vi "Add User.vi"(8 "error in (no error)":errorcluster, 9 "Data":T1={"Password"="", "Access"=enum."Guest", "Array of Permissions"=[]}, 10 "Username":string, 11 "UserPwd DB in":refnum<class "UserPwd DB.lvclass">) -> (0 "error out":errorcluster, 3 "UserPwd DB out":refnum<class "UserPwd DB.lvclass">)   [LabVIEW 2016, in "UserPwd DB.lvlib" / "UserPwd DB.lvclass"]
uses:
  <userlib>/Common Components/UserPwd DB/UserPwd DB/UserPwd DB.lvclass
  <userlib>/Common Components/UserPwd DB/UserPwd DB/Data input.ctl
  <userlib>/Common Components/UserPwd DB/UserPwd DB/Access Level.ctl
  <userlib>/Common Components/UserPwd DB/UserPwd DB/Data saved.ctl
  <userlib>/Common Components/UserPwd DB/UserPwd DB/UserPwd DB.lvclass/UserPwd DB.ctl
  <vilib>/Utility/error.llb/Error Cluster From Error Code.vi
  <vilib>/ErrorRing/Error Ring.xnode
  <vilib>/addons/_JKI.lib/Serialization/JSON/JKI JSON Serialization.lvlib
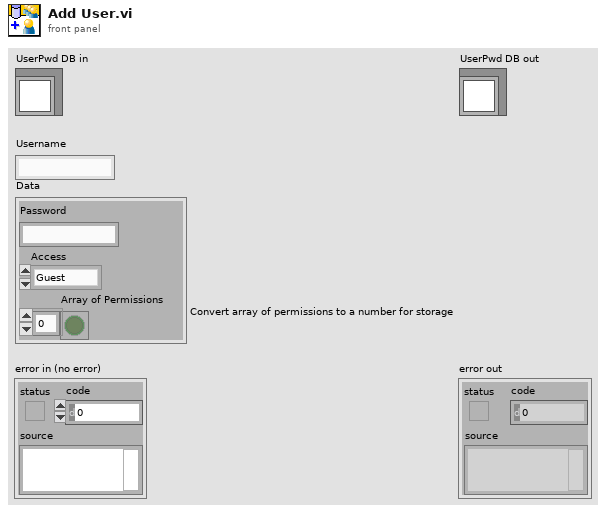
[diagram p1: front panel]
types:
  T1 = typedef "UserPwd DB.lvlib/UserPwd DB.lvclass/Data input.ctl" = cluster{"Password":string, "Access":T2, "Array of Permissions":bool[]}
  T2 = typedef "UserPwd DB.lvlib/UserPwd DB.lvclass/Access Level.ctl" = enum16{"Admin", "User lv1", "User lv2", "User lv3", "User lv4", "User lv5", "User lv6", "User lv7", "User lv8", "User lv9", "Guest"}
  T3 = typedef "UserPwd DB.lvlib/UserPwd DB.lvclass/Data saved.ctl" = cluster{"Encrypted Password":string, "Access":T2, "Permission":u32}
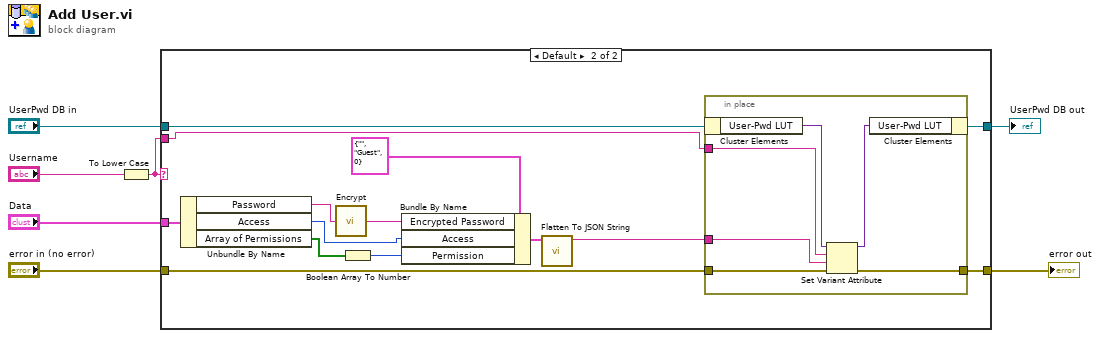
[diagram p0: block diagram]
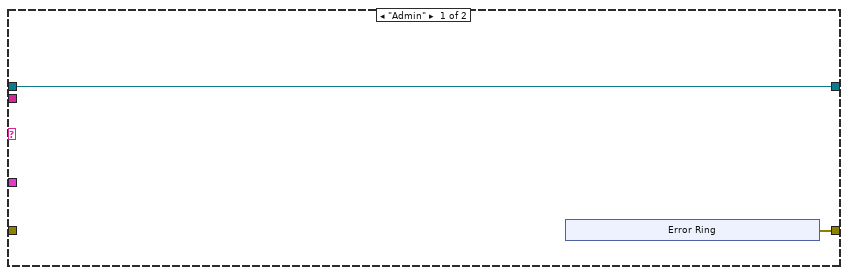
[diagram p2: hidden frame]
diagram:
  n1 = To Lower Case(string="Username") -> (all lower case string=w1:string)
  n2 = case shown="Default" w1 {
    tunnel: "UserPwd DB in" -> [w9 w27]
    tunnel: [w9 w26] -> w6
    tunnel: w1 -> [_ w25]
    tunnel: "error in (no error)" -> [_ w23]
    tunnel: [w8 w22] -> w4
    tunnel: "Data" -> [_ w21]
    frame "Admin" {
      n3 = xnode "Error Ring"() -> ("error out"=w8:errorcluster)
    }
    frame Default {
      n4 = Unbundle By Name(w21) -> ("Password"=w19:string, "Access"=w16:T2, "Array of Permissions"=w15:bool[])
      n5 = call <userlib>:"Encrypt.vi"("String"=w19) -> ("Encrypted String"=w18:string)
      n6 = Boolean Array To Number(Boolean array=w15) -> (number=w14:u32)
      n7 = Bundle By Name(cluster=T3 {"Encrypted Password"="", "Access"=enum."Guest", "Permission"=0} ("Data"), "Encrypted Password"=w18, "Access"=w16, "Permission"=w14) -> (w20:T3)
      n8 = call <vilib>:"Flatten To JSON String.vi"("Variant"=w20) -> ("JSON String"=w24:string)  [unwired: 9 in, 1 out]
      n9 = in-place {
        in-place-border: w25 -> [w31]
        in-place-border: w24 -> [w30]
        in-place-border: w23 -> [w29]
        in-place-border: [w28] -> w22
        n10 = in-place-cluster #1(w27) -> ("User-Pwd LUT"=w33:variant)
        n11 = Set Variant Attribute(Variant=w33, name=w31, value=w30, error in=w29) -> (Variant out=w32:variant, error out=w28:errorcluster)  [unwired: 1 out]
        n12 = in-place-cluster #1("User-Pwd LUT"=w32) -> (w26:refnum<class "UserPwd DB.lvclass">)
      }
    }
  }
  "error out" <- w4
  "UserPwd DB out" <- w6
